vi "PowerElectrodesDlg.vi"(8 "error in":errorcluster caption="error out") -> (0 "error out":errorcluster)   [LabVIEW 2014, in "PowerElectrodes.lvlib"]
uses:
  PowerElectrodes.lvlib
  <vilib>/Utility/miscctls.llb/LVRowAndColumnTypeDef.ctl
  DataBase/DataBase.lvlib
  DetectElecrodes/DetectElectros.lvlib
panel:
  in  "退出":bool
  in  "删除":bool
  in  "修改":bool
  in  "新增":bool
  in  "供电电极管理":i32(listbox)
  in  "OK":bool
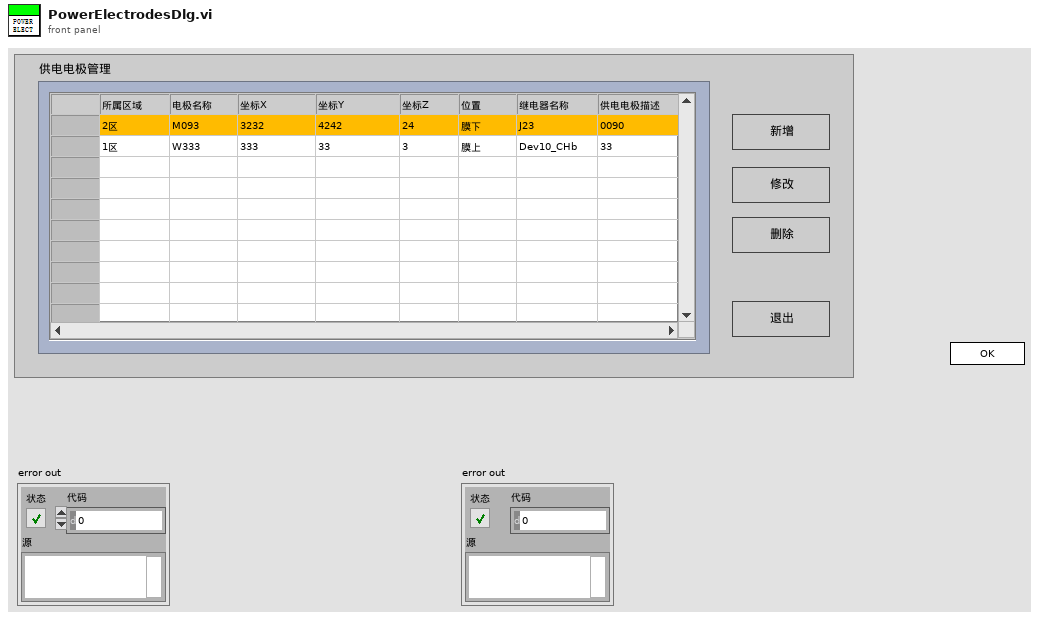
[diagram p1: front panel]
types:
  T1 = enum32{"invalid app kind", "Development System", "Run Time System", "Student Edition", "Embedded LabVIEW", "Evaluation", "Custom"}
  T2 = enum32{"Invalid", "Standard", "Closed", "Hidden", "Minimized", "Maximized"}
  T3 = typedef "LVPoint32TypeDef.ctl" = cluster{"Horizontal":i32, "Vertical":i32}
  T4 = typedef "LVRowAndColumnTypeDef.ctl" = cluster{"Row":i32, "Column":i32}
  T5 = cluster{"Core":cluster{"Current VI Reference":refnum<vi>, "Close Panel on Exit?":bool}, "Your Boolean data":bool, "Your string data":string, "DataP_Init":cluster{i32, "电极名称":string, "区域名称":string, "坐标X":string, "坐标Y":string, "坐标Z":string, "电极位置":string, "继电器名称":string, "继电器极性":string, "电极描述":string}, "行列编号":T4}
  T6 = cluster{i32, "电极名称":string, "区域名称":string, "坐标X":string, "坐标Y":string, "坐标Z":string, "电极位置":string, "继电器名称":string, "继电器极性":string, "电极描述":string}
  T7 = cluster{"Current VI Reference":refnum<vi>, "Close Panel on Exit?":bool}
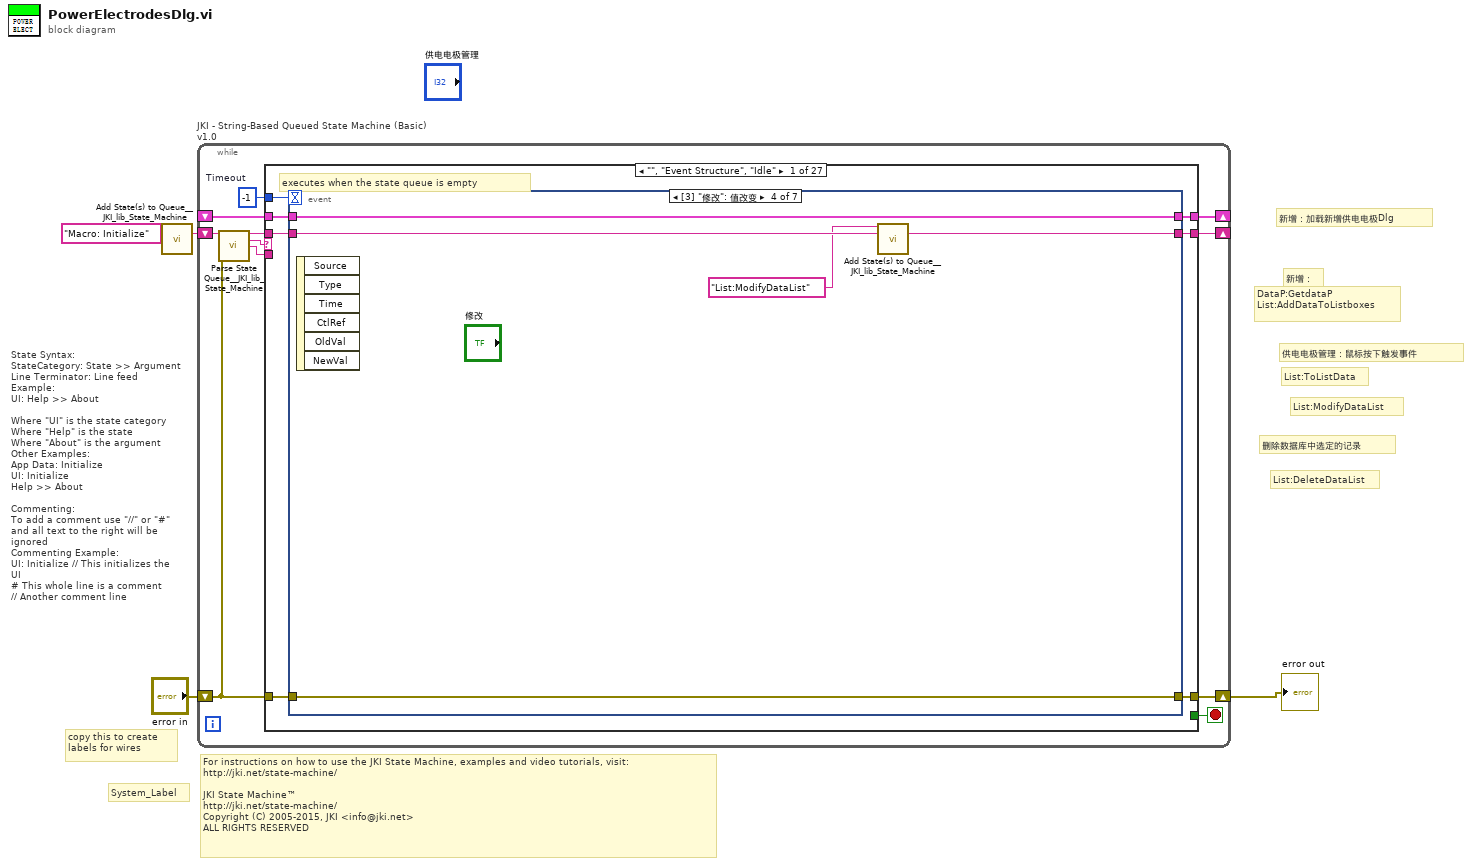
[diagram p0: block diagram]
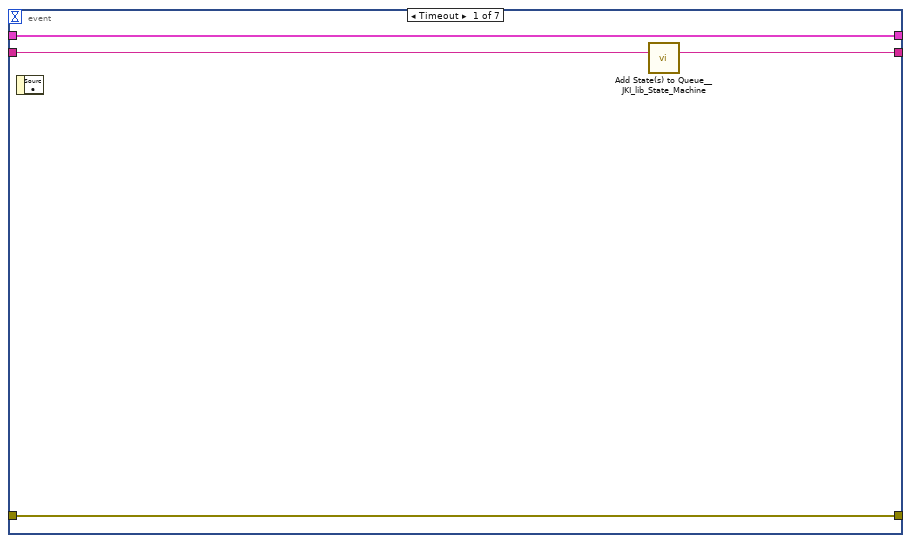
[diagram p2: hidden frame]
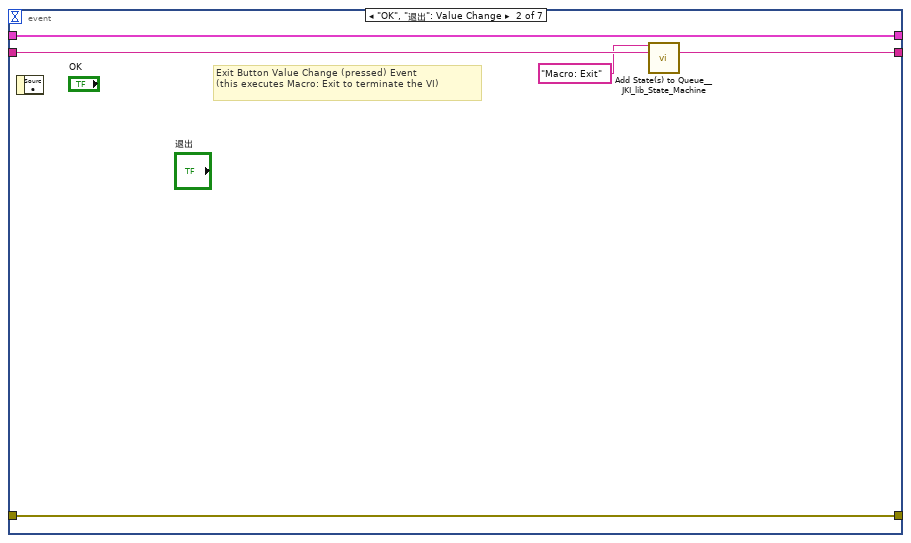
[diagram p3: hidden frame]
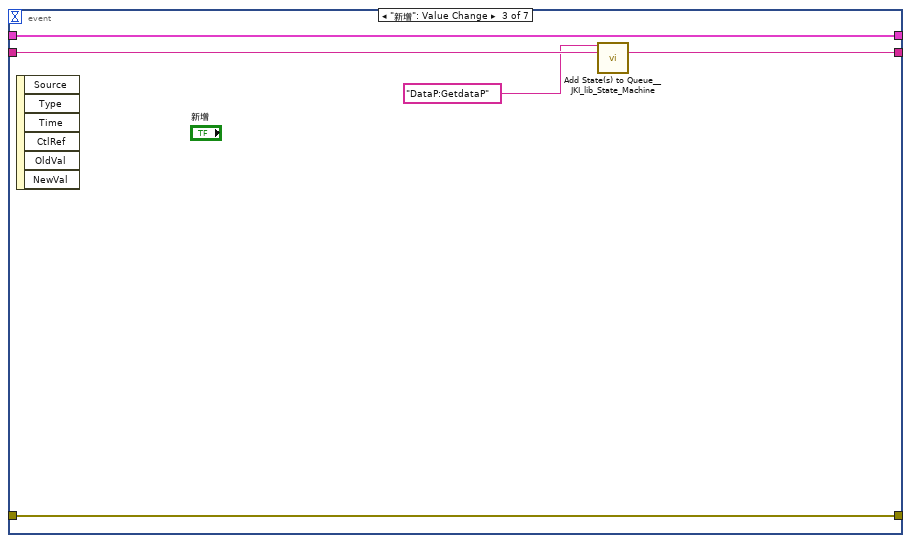
[diagram p4: hidden frame]
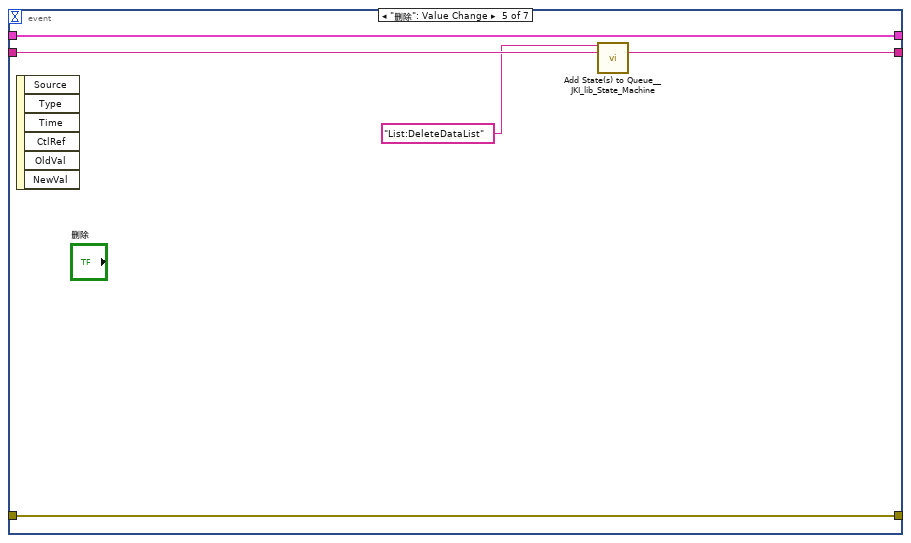
[diagram p5: hidden frame]
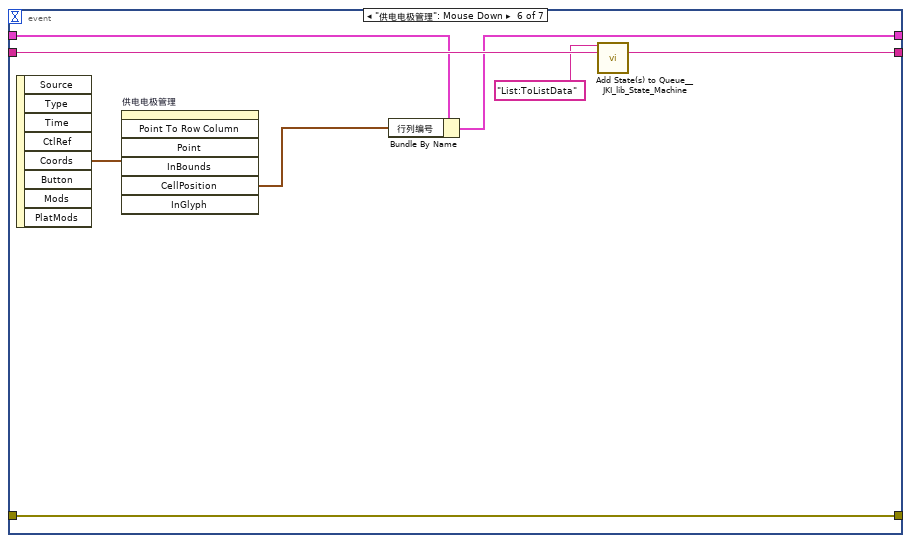
[diagram p6: hidden frame]
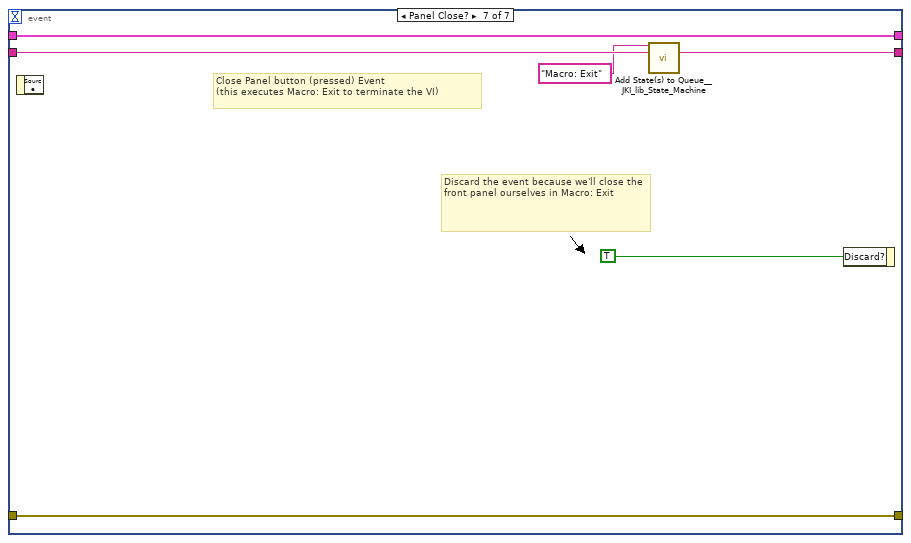
[diagram p7: hidden frame]
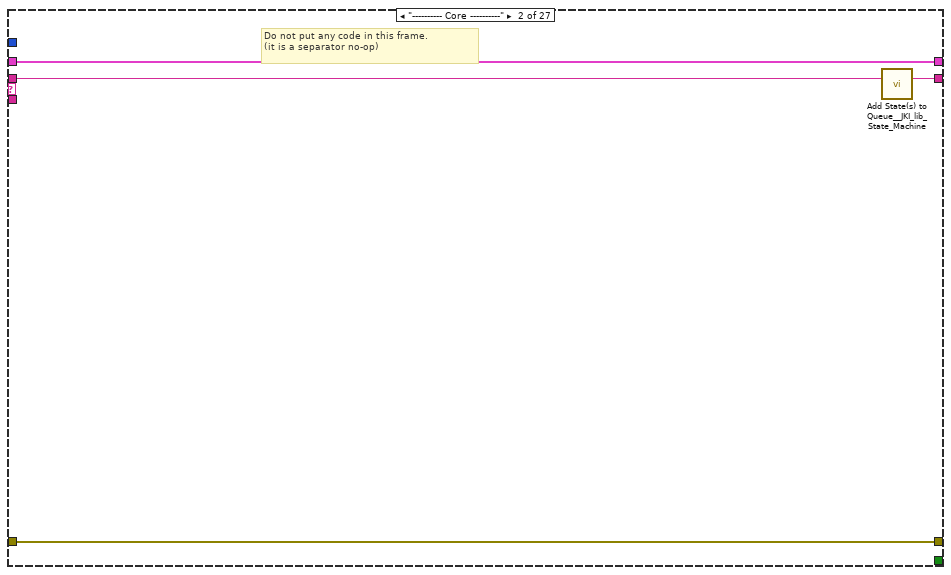
[diagram p8: hidden frame]
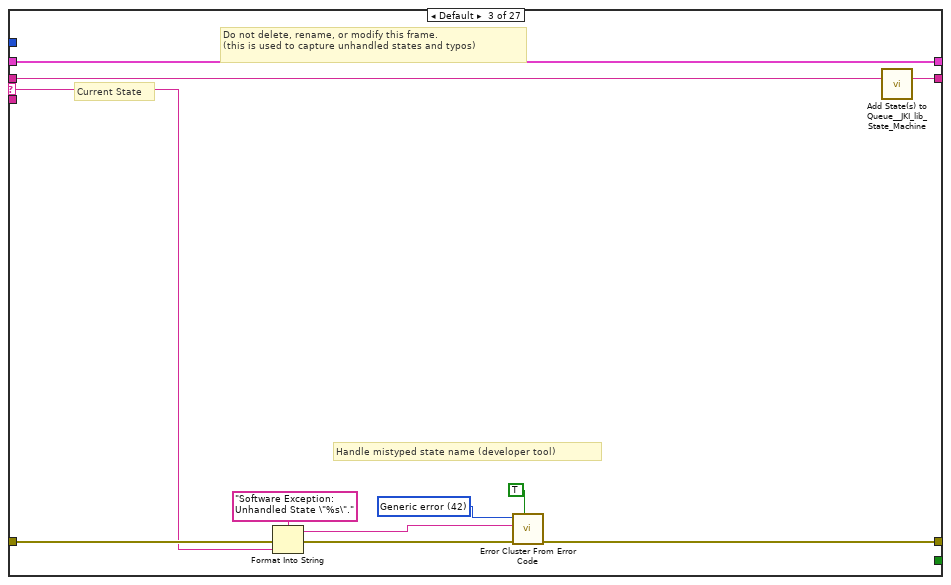
[diagram p9: hidden frame]
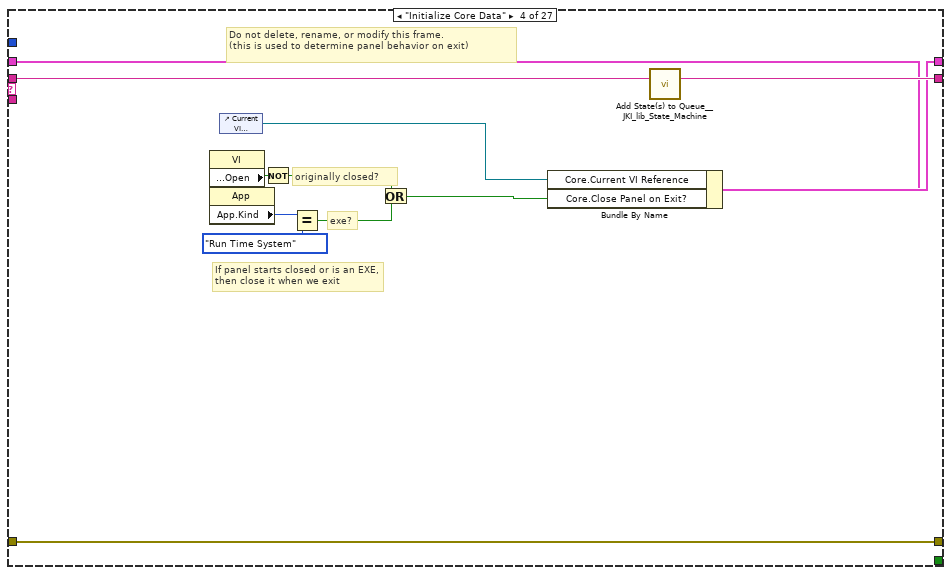
[diagram p10: hidden frame]
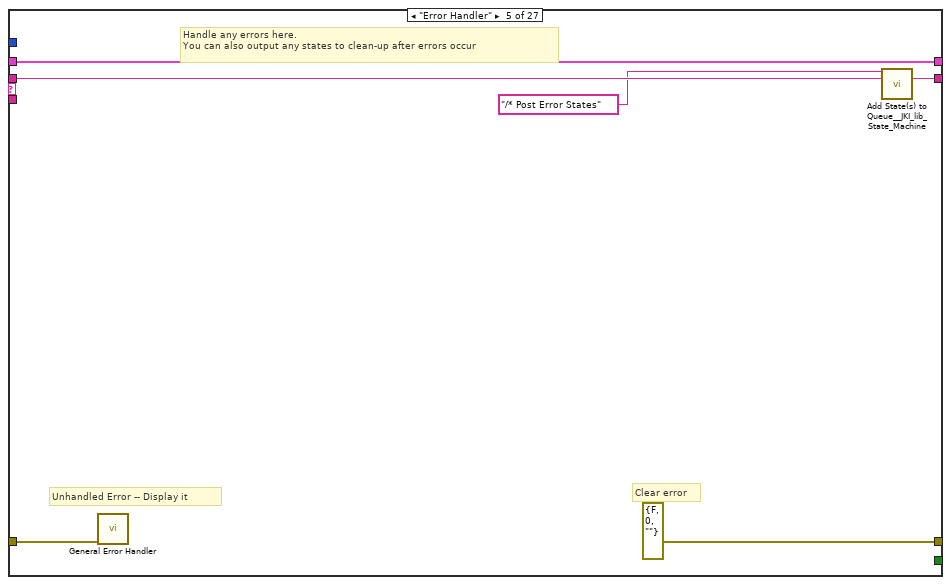
[diagram p11: hidden frame]
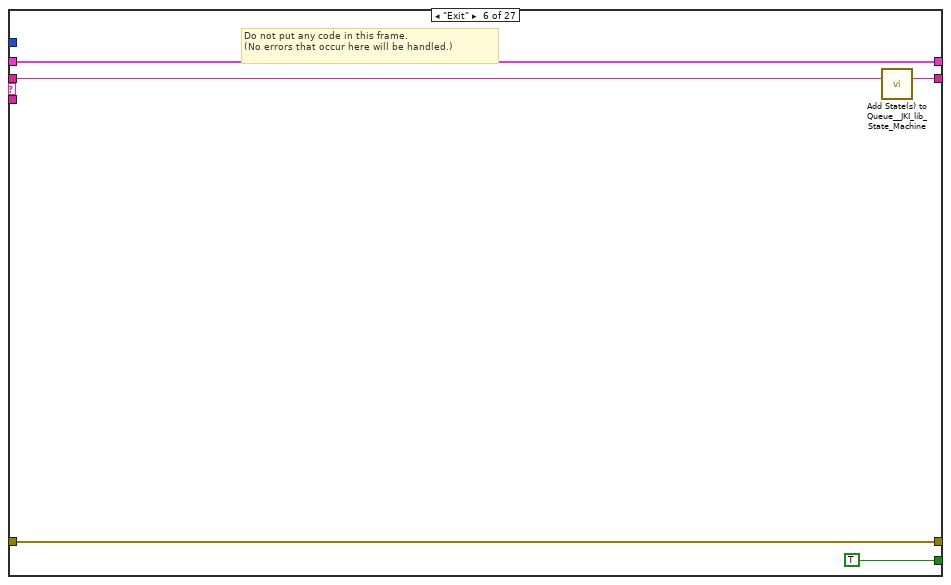
[diagram p12: hidden frame]
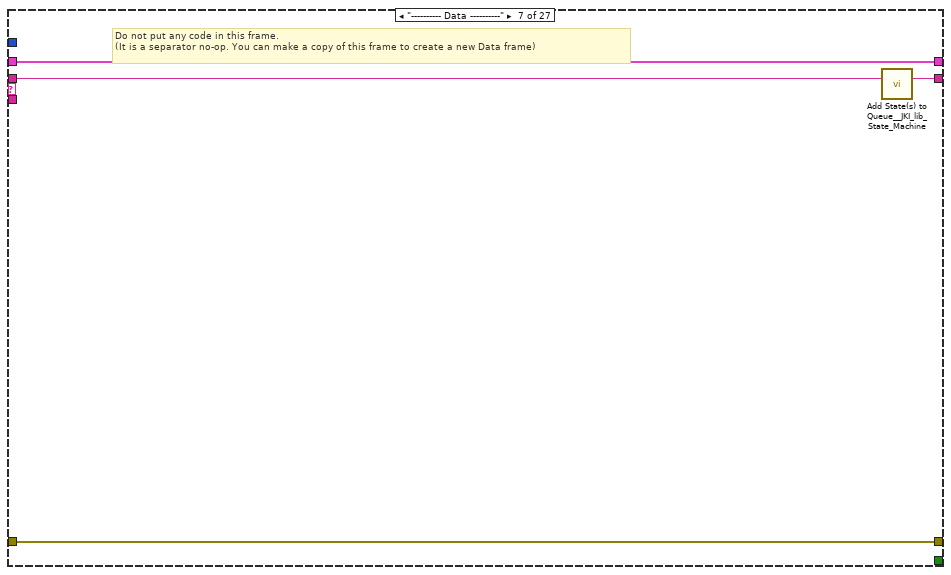
[diagram p13: hidden frame]
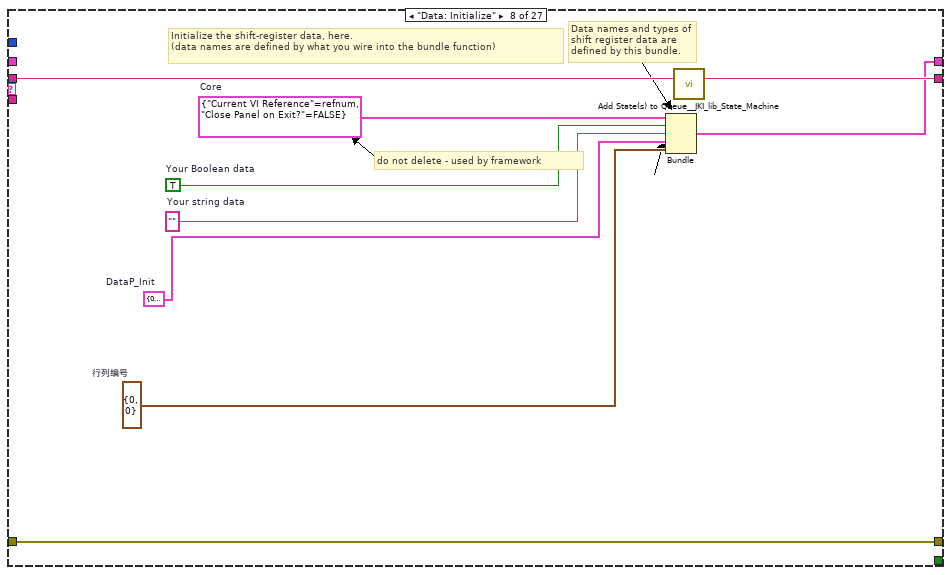
[diagram p14: hidden frame]
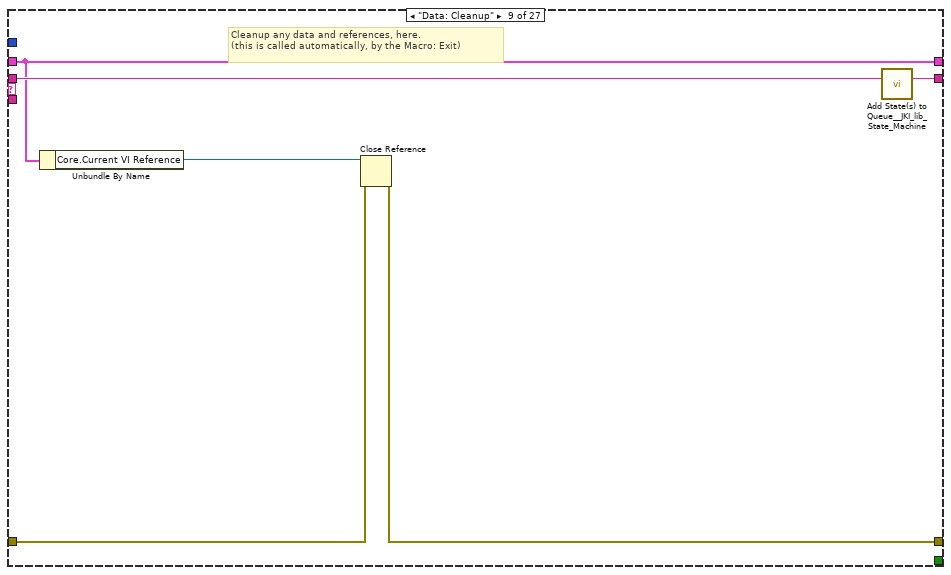
[diagram p15: hidden frame]
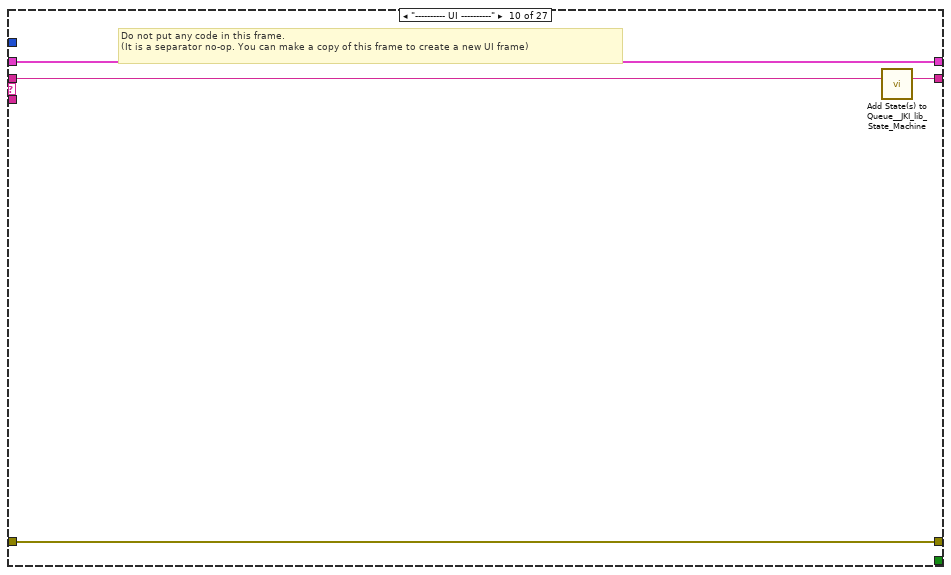
[diagram p16: hidden frame]
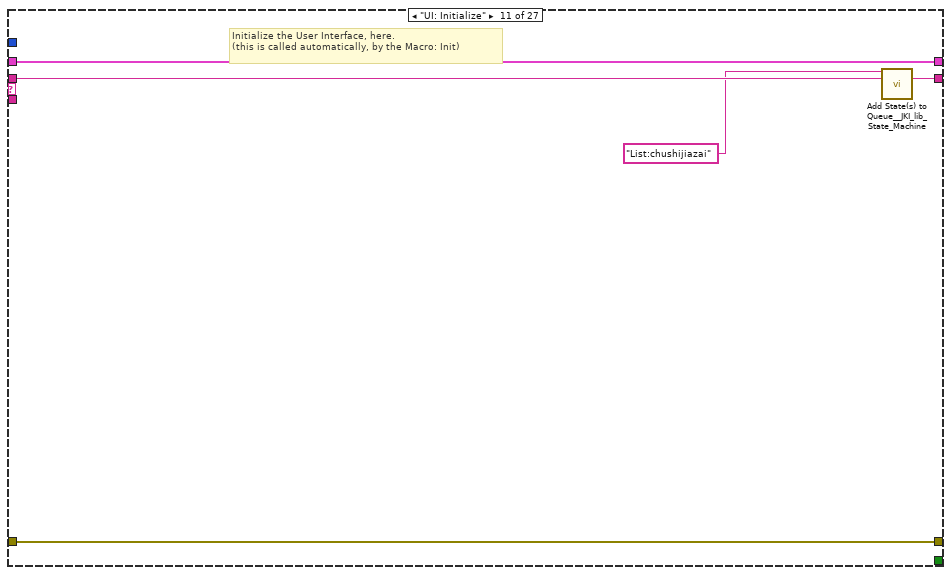
[diagram p17: hidden frame]
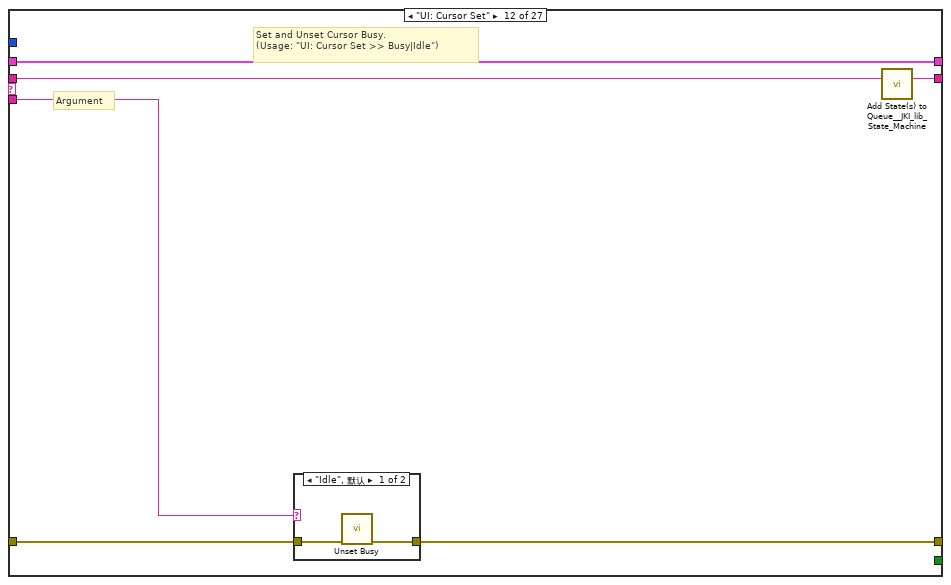
[diagram p18: hidden frame]
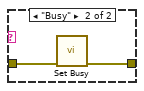
[diagram p19: hidden frame]
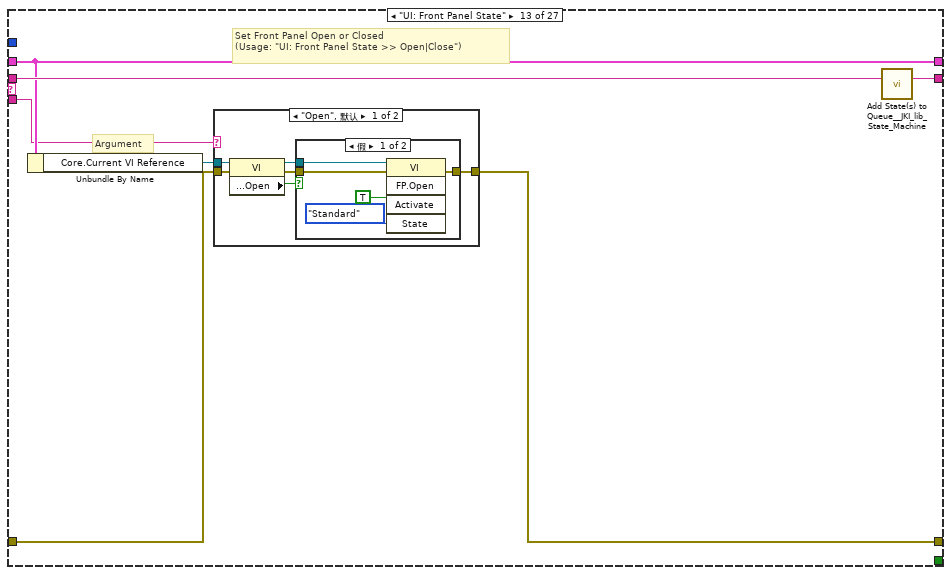
[diagram p20: hidden frame]
diagram:
  # "List:DeleteDataList"
  # "删除数据库中选定的记录"
  # "List:ModifyDataList"
  # "List:ToListData"
  # "供电电极管理：鼠标按下触发事件"
  # "新增："
  # "DataP:GetdataP\nList:AddDataToListboxes"
  # "新增：加载新增供电电极Dlg"
  # "For instructions on how to use the JKI State Machine, examples and video tutorials, visit:\nhttp://jki.net/state-machine/\n\nJKI State Machine™\nhttp://jki.net/state-machine/\nCopyright (C) 2005-2015, JKI <info@jki.net>\nALL RIGHTS RESERVED"
  # "State Syntax:\nStateCategory: State >> Argument\nLine Terminator: Line feed\nExample:\nUI: Help >> About\n\nWhere \"UI\" is the state category\nWhere \"Help\" is the state\nWhere \"About\" is the argument\nOther Examples:\nApp Data: Initialize\nUI: Initialize\nHelp >> About\n\nCommenting:\nTo add a comment use \"//\" or \"#\" and all text to the right will be ignored\nCommenting Example:\nUI: Initialize // This initializes the UI\n# This whole line is a comment\n// Another comment line"
  # "copy this to create labels for wires"
  # "System_Label"
  n1 = call <vilib>:"Add State(s) to Queue__JKI_lib_State_Machine.vi"("State(s) in (\"\")"="Macro: Initialize") -> ("States Out"=w4:string)  [unwired: 14 in]
  n2 = while "JKI - String-Based Queued State Machine (Basic) v1.0" {
    shift-right: [w8] -> _
    shift-left: _ -> [w7]
    shift-right: [w11] -> w2
    shift-left: "error in" -> [w5]
    shift-right: [w10] -> _
    shift-left: w4 -> [w12]
    stop <- w9 stop-if-true
    w6 = -1  # Timeout
    n3 = call <vilib>:"Parse State Queue__JKI_lib_State_Machine.vi"("State Queue"=w12, "Error In (no error)"=w5) -> ("Remaining States"=w14:string, "Current State"=w15:string, "Arguments"=w13:string)  [unwired: 11 in]
    n4 = case shown="\"\", \"Event Structure\", \"Idle\"" w15 {
      selector: w15 -> [_ _ w65 _ _ _ _ _ _ _ _ _ _ _ _ _ _ _ _ _ _ _ _ _ _ _ _]
      tunnel: w14 -> [w22 w64 w69 w87 w93 w98 w102 w111 w117 w121 w126 w132 w143 w169 w174 w184 w188 w192 w201 w208 w212 w225 w252 w279 w283 w287 w291]
      tunnel: w13 -> [_ _ _ _ _ _ _ _ _ _ _ w127 w137 _ _ _ _ _ _ _ _ _ _ _ _ _ _]
      tunnel: w7 -> [w20 w61 w67 w78 w90 w96 w99 _ w112 w118 w124 w130 w139 w166 w171 w181 w185 w189 w198 w204 w209 w222 w249 w276 w280 w284 w288]
      tunnel: [w19 w62 w71 w84 errorcluster {"status"=FALSE, "code"=0, "source"=""} ("error out") w95 w100 w108 w113 w119 w123 w128 w140 w167 w172 w182 w186 w190 w199 w206 w210 w223 w250 w277 w281 w285 w289] -> w11
      tunnel: w5 -> [w18 w62 w70 w84 w89 w95 w100 w108 w114 w119 w123 w129 w141 w167 w172 w182 w186 w190 w199 w206 w210 w223 w250 w277 w281 w285 w289]
      tunnel: [w21 w63 w68 w86 w92 w97 w101 w110 w116 w120 w125 w131 w142 w168 w173 w183 w187 w191 w200 w207 w211 w224 w251 w278 w282 w286 w290] -> w10
      tunnel: [_ _ _ _ _ TRUE _ _ _ _ _ _ _ _ _ _ _ _ _ _ _ _ _ _ _ _ _] -> w9
      tunnel: [w17 w61 w67 w85 w90 w96 w99 w109 w112 w118 w124 w130 w139 w166 w171 w181 w185 w189 w198 w203 w209 w222 w249 w276 w280 w284 w288] -> w8
      tunnel: w6 -> [w16 _ _ _ _ _ _ _ _ _ _ _ _ _ _ _ _ _ _ _ _ _ _ _ _ _ _]
      frame "", "Event Structure", "Idle" {
        # "executes when the state queue is empty"
        n5 = event shown="[3] \"修改\": 值改变" {
          selector: _ -> [_ _ _ _ _ _ _]
          dyn-events: _ -> [_ _ _ _ _ _ _]
          timeout: w16 -> [_ _ _ _ _ _ _]
          tunnel: w22 -> [w26 w31 w34 w39 w44 w53 w60]
          tunnel: [w25 w30 w35 w40 w45 w54 w59] -> w21
          tunnel: w20 -> [w23 w28 w36 w41 w46 w49 w57]
          tunnel: [w24 w29 w33 w38 w43 w52 w58] -> w19
          tunnel: w18 -> [w24 w29 w33 w38 w43 w52 w58]
          tunnel: [w23 w28 w36 w41 w46 w48 w57] -> w17
          event Timeout {
            n6 = event-data() -> ()  [unwired: 1 in, 1 out]
            n7 = call <vilib>:"Add State(s) to Queue__JKI_lib_State_Machine.vi"("State(s) in (\"\")"=w26) -> ("States Out"=w25:string)  [unwired: 14 in]
          }
          event "OK", "退出": Value Change {
            # "Exit Button Value Change (pressed) Event\n(this executes Macro: Exit to terminate the VI)"
            n8 = event-data() -> ()  [unwired: 1 in, 1 out]
            n9 = call <vilib>:"Add State(s) to Queue__JKI_lib_State_Machine.vi"("State(s) in Front (\"\")"="Macro: Exit", "State(s) in (\"\")"=w31) -> ("States Out"=w30:string)  [unwired: 13 in]
          }
          event "新增": Value Change {
            n10 = event-data() -> ()  [unwired: 1 in, 6 out]
            n11 = call <vilib>:"Add State(s) to Queue__JKI_lib_State_Machine.vi"("State(s) in Front (\"\")"="DataP:GetdataP", "State(s) in (\"\")"=w34) -> ("States Out"=w35:string)  [unwired: 13 in]
          }
          event "修改": Value Change {
            n12 = event-data() -> ()  [unwired: 1 in, 6 out]
            n13 = call <vilib>:"Add State(s) to Queue__JKI_lib_State_Machine.vi"("State(s) in Front (\"\")"="List:ModifyDataList", "State(s) in (\"\")"=w39) -> ("States Out"=w40:string)  [unwired: 13 in]
          }
          event "删除": Value Change {
            n14 = event-data() -> ()  [unwired: 1 in, 6 out]
            n15 = call <vilib>:"Add State(s) to Queue__JKI_lib_State_Machine.vi"("State(s) in Front (\"\")"="List:DeleteDataList", "State(s) in (\"\")"=w44) -> ("States Out"=w45:string)  [unwired: 13 in]
          }
          event "供电电极管理": Mouse Down {
            n16 = event-data() -> ("Coords"=w51:T3)  [unwired: 1 in, 7 out]
            n17 = invoke on="供电电极管理" class="MCListbox (严格)" method="Point To Row Column"("Point"=w51) -> ("CellPosition"=w50:T4)  [unwired: 6 in, 6 out]
            n18 = Bundle By Name(cluster=w49, "行列编号"=w50) -> (w48:T5)
            n19 = call <vilib>:"Add State(s) to Queue__JKI_lib_State_Machine.vi"("State(s) in Front (\"\")"="List:ToListData", "State(s) in (\"\")"=w53) -> ("States Out"=w54:string)  [unwired: 13 in]
          }
          event Panel Close? {
            # "Discard the event because we'll close the front panel ourselves in Macro: Exit"
            # "Close Panel button (pressed) Event\n(this executes Macro: Exit to terminate the VI)"
            n20 = event-data() -> ()  [unwired: 1 in, 1 out]
            n21 = call <vilib>:"Add State(s) to Queue__JKI_lib_State_Machine.vi"("State(s) in Front (\"\")"="Macro: Exit", "State(s) in (\"\")"=w60) -> ("States Out"=w59:string)  [unwired: 13 in]
            n22 = event-data("Discard?"=TRUE) -> ()  [unwired: 1 in, 1 out]
          }
        }
      }
      frame "---------- Core ----------" {
        # "Do not put any code in this frame.\n(it is a separator no-op)"
        n23 = call <vilib>:"Add State(s) to Queue__JKI_lib_State_Machine.vi"("State(s) in (\"\")"=w64) -> ("States Out"=w63:string)  [unwired: 14 in]
      }
      frame Default {
        w74 = 42 items=["No error", "Argument error", "Memory is full", "Out of zone", "End of file", "File already open", "Generic file I/O error", "File not found", "File permission error", "Disk is full", "Duplicate path", "Too many files open", "System feature not enabled", "Resource file not found", "Cannot add resource", "Resource not found", "Image not found", "Image memory error", "Pen does not exist", "Config type invalid", "Config token not found", "Config parse error", "Config memory error", "Bad external code format", "Bad external code offset", "External code not present", "Null window", "Destroy window error", "Null menu", "Print aborted", "Bad print record", "Print driver error", "Windows error during printing", "Memory error during printing", "Print dialog error", "Generic print error", "Invalid device refnum", "Device not found", "Device parameter error", "Device unit error", "Cannot open device", "Device call aborted", "Generic error", "Cancelled by user", "Object ID too low", "Object ID too high", "Object not in heap", "Unknown heap", "Unknown object (invalid DefProc)", "Unknown object (DefProc not in table)", "Message out of range", "Invalid (null) method", "Unknown message", "Manager call not supported", "Bad address", "Network operation in progress", "Network operation timed out", "Connection is busy", "Network attribute not supported", "Network error", "Address in use", "System out of memory", "Connection aborted", "Connection refused", "Not connected", "Already connected", "Connection closed", "Initialization error (interapplication manager)", "Bad occurrence", "Wait on unbound occurrence handler", "Occurrence queue overflow", "Datalog type conflict", "Unused", "Unrecognized type (interapplication manager)", "Memory corrupt", "Failed to make temporary DLL", "Old CIN version", "Drag socket not found", "Failed to load drop-object", "Failed to register OLE object", "Failed to release OLE object", "Format specifier type mismatch", "Unknown format specifier", "Too few format specifiers", "Too many format specifiers", "Scan failed", "Newer CIN version", "Error converting to variant", "Runtime menu error", "Password tampered", "Variant attribute not found", "Incompatible variant data type", "Event data is not available", "Event Store is not present", "Occurrence is not found", "Event Queue is not created", "Event info is not available", "Refnum passed is NULL", "Error retrieving Class GUID", "Error retrieving CoClass GUID", "Error retrieving TypeLib GUID.", "Bad built application magic bytes.", "Specific driver is different from the specific driver associated with the Logical Name.", "There is no session opened to the class driver.", "Max Error", "MAX - Error with config objects", "MAX - Error loading configuration", "MAX - Group not supported"]
        # "Current State"
        # "Do not delete, rename, or modify this frame.\n(this is used to capture unhandled states and typos)"
        # "Handle mistyped state name (developer tool)"
        n24 = Format Into String(format string="Software Exception: Unhandled State \"%s\"." ("message"), error in=w70, w65) -> (resulting string=w73:string, error out=w72:errorcluster)  [unwired: 1 in]
        n25 = call <vilib>:"Error Cluster From Error Code.vi"("show call chain? (False)"=TRUE, "error in (no error)"=w72, "error message (\"\")"=w73, "error code (0)"=w74) -> ("error out"=w71:errorcluster)  [unwired: 5 in]
        n26 = call <vilib>:"Add State(s) to Queue__JKI_lib_State_Machine.vi"("State(s) in (\"\")"=w69) -> ("States Out"=w68:string)  [unwired: 14 in]
      }
      frame "Initialize Core Data" {
        # "Do not delete, rename, or modify this frame.\n(this is used to determine panel behavior on exit)"
        # "originally closed?"
        # "exe?"
        # "If panel starts closed or is an EXE, then close it when we exit"
        n27 = property class="VI"() -> ("Front Panel.Open"=w83:bool)  [unwired: 2 in, 2 out]
        n28 = property class="App"() -> ("App.Kind"=w82:T1)  [unwired: 2 in, 2 out]
        n29 = control-ref of="Current VI Reference"() -> (w76:refnum<vi>)
        n30 = Not(x=w83) -> (.not. x?=w80:bool)
        n31 = Equal?(x=w82, y=T1."Run Time System" ("Application:Kind")) -> (x = y?=w79:bool)
        n32 = Or(x=w80, y=w79) -> (x .or. y?=w77:bool)
        n33 = Bundle By Name(cluster=w78, "Core.Current VI Reference"=w76, "Core.Close Panel on Exit?"=w77) -> (w85:T5)
        n34 = call <vilib>:"Add State(s) to Queue__JKI_lib_State_Machine.vi"("State(s) in (\"\")"=w87) -> ("States Out"=w86:string)  [unwired: 14 in]
      }
      frame "Error Handler" {
        # "Unhandled Error -- Display it"
        # "Handle any errors here.\nYou can also output any states to clean-up after errors occur"
        # "Clear error"
        n35 = call <vilib>:"General Error Handler.vi"("error in (no error)"=w89) -> ()  [unwired: 10 in, 5 out]
        n36 = call <vilib>:"Add State(s) to Queue__JKI_lib_State_Machine.vi"("State(s) in Front (\"\")"="/* Post Error States", "State(s) in (\"\")"=w93) -> ("States Out"=w92:string)  [unwired: 13 in]
      }
      frame "Exit" {
        # "Do not put any code in this frame.\n(No errors that occur here will be handled.)"
        n37 = call <vilib>:"Add State(s) to Queue__JKI_lib_State_Machine.vi"("State(s) in (\"\")"=w98) -> ("States Out"=w97:string)  [unwired: 14 in]
      }
      frame "---------- Data ----------" {
        # "Do not put any code in this frame.\n(It is a separator no-op. You can make a copy of this frame to create a new Data frame)"
        n38 = call <vilib>:"Add State(s) to Queue__JKI_lib_State_Machine.vi"("State(s) in (\"\")"=w102) -> ("States Out"=w101:string)  [unwired: 14 in]
      }
      frame "Data: Initialize" {
        w103 = T4 {"Row"=0, "Column"=0}  # 行列编号
        w104 = T6 {0, "电极名称"="", "区域名称"="", "坐标X"="", "坐标Y"="", "坐标Z"="", "电极位置"="", "继电器名称"="", "继电器极性"="", "电极描述"=""}  # DataP_Init
        w105 = T7 {"Current VI Reference"=refnum, "Close Panel on Exit?"=FALSE}  # Core
        w107 = TRUE  # Your Boolean data
        w106 = ""  # Your string data
        # "do not delete - used by framework"
        # "Data names and types of shift register data are defined by this bundle."
        # "Initialize the shift-register data, here.\n(data names are defined by what you wire into the bundle function)"
        n39 = Bundle("Core"=w105, "Your Boolean data"=w107, "Your string data"=w106, "DataP_Init"=w104, "行列编号"=w103) -> (w109:T5)  [unwired: 1 in]
        n40 = call <vilib>:"Add State(s) to Queue__JKI_lib_State_Machine.vi"("State(s) in (\"\")"=w111) -> ("States Out"=w110:string)  [unwired: 14 in]
      }
      frame "Data: Cleanup" {
        # "Cleanup any data and references, here.\n(this is called automatically, by the Macro: Exit)"
        n41 = Unbundle By Name(w112) -> ("Core.Current VI Reference"=w115:refnum<vi>)
        n42 = Close Reference(reference=w115, error in (no error)=w114) -> (error out=w113:errorcluster)
        n43 = call <vilib>:"Add State(s) to Queue__JKI_lib_State_Machine.vi"("State(s) in (\"\")"=w117) -> ("States Out"=w116:string)  [unwired: 14 in]
      }
      frame "---------- UI ----------" {
        # "Do not put any code in this frame.\n(It is a separator no-op. You can make a copy of this frame to create a new UI frame)"
        n44 = call <vilib>:"Add State(s) to Queue__JKI_lib_State_Machine.vi"("State(s) in (\"\")"=w121) -> ("States Out"=w120:string)  [unwired: 14 in]
      }
      frame "UI: Initialize" {
        # "Initialize the User Interface, here.\n(this is called automatically, by the Macro: Init)"
        n45 = call <vilib>:"Add State(s) to Queue__JKI_lib_State_Machine.vi"("State(s) in Front (\"\")"="List:chushijiazai", "State(s) in (\"\")"=w126) -> ("States Out"=w125:string)  [unwired: 13 in]
      }
      frame "UI: Cursor Set" {
        # "Argument"
        # "Set and Unset Cursor Busy.\n(Usage: \"UI: Cursor Set >> Busy|Idle\")"
        n46 = case shown="\"Idle\", 默认" w127 {
          tunnel: w129 -> [w134 w136]
          tunnel: [w133 w135] -> w128
          frame "Idle", Default {
            n47 = call <vilib>:"Unset Busy.vi"("error in (no error)"=w134) -> ("error out"=w133:errorcluster)  [unwired: 10 in]
          }
          frame "Busy" {
            n48 = call <vilib>:"Set Busy.vi"("error in (no error)"=w136) -> ("error out"=w135:errorcluster)  [unwired: 9 in, 1 out]
          }
        }
        n49 = call <vilib>:"Add State(s) to Queue__JKI_lib_State_Machine.vi"("State(s) in (\"\")"=w132) -> ("States Out"=w131:string)  [unwired: 14 in]
      }
      frame "UI: Front Panel State" {
        # "Argument"
        # "Set Front Panel Open or Closed\n(Usage: \"UI: Front Panel State >> Open|Close\")"
        n50 = Unbundle By Name(w139) -> ("Core.Current VI Reference"=w138:refnum<vi>)
        n51 = case shown="\"Open\", 默认" w137 {
          tunnel: w141 -> [w147 w160]
          tunnel: [w149 w161] -> w140
          tunnel: w138 -> [w148 w158]
          frame "Open", Default {
            n52 = property class="VI"(reference=w148, error in=w147) -> (reference out=w145:refnum<vi>, error out=w146:errorcluster, "Front Panel.Open"=w144:bool)
            n53 = case shown="假" w144 {
              tunnel: [w152 w155] -> w149
              tunnel: w146 -> [w151 w155]
              tunnel: w145 -> [w150 _]
              frame False {
                n54 = invoke class="VI" method="FP.Open"(reference=w150, error in=w151, "Activate"=TRUE, "State"=T2."Standard") -> (error out=w152:errorcluster)  [unwired: 1 in, 4 out]
              }
              frame True {
              }
            }
          }
          frame "Close" {
            n55 = property class="VI"(reference=w158, error in=w160) -> (reference out=w157:refnum<vi>, error out=w159:errorcluster, "Front Panel.Open"=w156:bool)
            n56 = case shown="真" w156 {
              tunnel: [w162 w165] -> w161
              tunnel: w159 -> [w162 w164]
              tunnel: w157 -> [_ w163]
              frame False {
              }
              frame True {
                n57 = invoke class="VI" method="FP.Close"(reference=w163, error in=w164) -> (error out=w165:errorcluster)  [unwired: 1 in, 2 out]
              }
            }
          }
        }
        n58 = call <vilib>:"Add State(s) to Queue__JKI_lib_State_Machine.vi"("State(s) in (\"\")"=w143) -> ("States Out"=w142:string)  [unwired: 14 in]
      }
      frame "---------- Macro ----------" {
        # "Do not put any code in this frame.\n(It is a separator no-op. You can make a copy of this frame to create a new Macro frame)"
        n59 = call <vilib>:"Add State(s) to Queue__JKI_lib_State_Machine.vi"("State(s) in (\"\")"=w169) -> ("States Out"=w168:string)  [unwired: 14 in]
      }
      frame "Macro: Initialize" {
        w170 = "Data: Initialize\nInitialize Core Data\nUI: Initialize\nUI: Front Panel State >> Open"  # Data: Initialize Initialize Core Data UI: Initialize UI: Front Panel State >> Open
        # "Initialization Macro\n(This is called once, when the VI starts)"
        n60 = call <vilib>:"Add State(s) to Queue__JKI_lib_State_Machine.vi"("State(s) in Front (\"\")"=w170, "State(s) in (\"\")"=w174) -> ("States Out"=w173:string)  [unwired: 13 in]
      }
      frame "Macro: Exit" {
        # "Exit Macro\n(This is called once, when the VI exits)"
        n61 = Unbundle By Name(w181) -> ("Core.Close Panel on Exit?"=w180:bool)
        n62 = Select(t="UI: Front Panel State >> Close", s=w180, f="") -> (s? t:f=w177:string)
        n63 = call <vilib>:"Add State(s) to Queue__JKI_lib_State_Machine.vi"("State(s) in (\"\")"=w177, "State(s) at Back (\"\")"="Data: Cleanup\nExit") -> ("States Out"=w175:string)  [unwired: 13 in]
        n64 = call <vilib>:"Add State(s) to Queue__JKI_lib_State_Machine.vi"("State(s) in Front (\"\")"=w175, "State(s) in (\"\")"=w184) -> ("States Out"=w183:string)  [unwired: 13 in]
      }
      frame "-----------DataP-----------" {
        # "Template Separator\n(You can make a copy of, or modify, this frame)"
        n65 = call <vilib>:"Add State(s) to Queue__JKI_lib_State_Machine.vi"("State(s) in (\"\")"=w188) -> ("States Out"=w187:string)  [unwired: 14 in]
      }
      frame "List:ToListData" {
        # "Template Separator\n(You can make a copy of, or modify, this frame)"
        n66 = call <vilib>:"Add State(s) to Queue__JKI_lib_State_Machine.vi"("State(s) in (\"\")"=w192) -> ("States Out"=w191:string)  [unwired: 14 in]
      }
      frame "List:DeleteDataList" {
        # "select power_electrodes_Id from t_power_electrodes  limit %s,1"
        # "Template Separator\n(You can make a copy of, or modify, this frame)"
        n67 = Unbundle By Name(w198) -> ("行列编号.Row"=w196:i32)
        n68 = Number To Decimal String(number=w196) -> (decimal integer string=w195:string)  [unwired: 1 in]
        n69 = Format Into String(format string="delete from t_power_electrodes where power_electrodes_id =(select tp.power_electrodes_id from \n(select power_electrodes_id from t_power_electrodes  limit %s,1) tp);", w195) -> (resulting string=w194:string)  [unwired: 2 in, 1 out]
        n70 = call "deleteData.vi"("SQL query"=w194) -> ()  [unwired: 10 in, 1 out]
        n71 = call <vilib>:"Add State(s) to Queue__JKI_lib_State_Machine.vi"("State(s) in Front (\"\")"="List:AddDataToListboxes", "State(s) in (\"\")"=w201) -> ("States Out"=w200:string)  [unwired: 13 in]
      }
      frame "DataP:GetdataP" {
        # "Template Separator\n(You can make a copy of, or modify, this frame)"
        n72 = call "New_Power_ElectrodesDlg.vi"() -> ("DataP"=w205:T6)  [unwired: 10 in, 1 out]
        n73 = Bundle By Name(cluster=w204, "DataP_Init"=w205) -> (w203:T5)
        n74 = call <vilib>:"Add State(s) to Queue__JKI_lib_State_Machine.vi"("State(s) in Front (\"\")"="List:AddDataToListboxes", "State(s) in (\"\")"=w208) -> ("States Out"=w207:string)  [unwired: 13 in]
      }
      frame "----------List-------" {
        # "Template Separator\n(You can make a copy of, or modify, this frame)"
        n75 = call <vilib>:"Add State(s) to Queue__JKI_lib_State_Machine.vi"("State(s) in (\"\")"=w212) -> ("States Out"=w211:string)  [unwired: 14 in]
      }
      frame "List:ModifyDataList" {
        # "Template Separator\n(You can make a copy of, or modify, this frame)"
        n76 = Unbundle By Name(w222) -> ("行列编号.Row"=w220:i32)
        n77 = Number To Decimal String(number=w220) -> (decimal integer string=w219:string)  [unwired: 1 in]
        n78 = Format Into String(format string="select *from t_power_electrodes limit %s,1", w219) -> (resulting string=w218:string)  [unwired: 2 in, 1 out]
        n79 = call "SelectData.vi"("SQL query"=w218) -> ("recordset data"=w217:variant[][])  [unwired: 7 in, 1 out]
        n80 = call "ReadDataFromDatabase.vi"("长度"=10, "index"=0, "recordset data"=w217) -> ("一行记录"=w214:string[])  [unwired: 7 in, 1 out]
        n81 = call "Modify_Power_ElectrodesDlg.vi"("一行记录"=w214) -> ()  [unwired: 8 in, 1 out]
        n82 = call <vilib>:"Add State(s) to Queue__JKI_lib_State_Machine.vi"("State(s) in Front (\"\")"="List:AddDataToListboxes", "State(s) in (\"\")"=w225) -> ("States Out"=w224:string)  [unwired: 13 in]
      }
      frame "List:AddDataToListboxes" {
        w238 = 1 ("索引")
        # "从数据库中更新List中数据"
        # "从数据库中获取再在List中显示，这样更新比较好"
        # "Template Separator\n(You can make a copy of, or modify, this frame)"
        n83 = call "SelectData.vi"("SQL query"="select *from t_power_electrodes") -> ("recordset data"=w247:variant[][])  [unwired: 7 in, 1 out]
        n84 = call "ReadDataFromDatabase.vi"("长度"=9, "index"=1, "recordset data"=w247) -> ("所有记录"=w234:string[][])  [unwired: 7 in, 1 out]
        n85 = Array Subset(array=w234, index (col)=w238, length (col)=w238) -> (w236:string[][])  [unwired: 2 in]
        n86 = Array Subset(array=w234, index (col)=0 ("索引"), length (col)=1 ("长度")) -> (w240:string[][])  [unwired: 2 in]
        n87 = Array Subset(array=w234, index (col)=2 ("索引")) -> (w241:string[][])  [unwired: 3 in]
        n88 = Array Subset(array=w234, index (col)=8, length (col)=1 ("索引")) -> (w230:string[][])  [unwired: 2 in]
        n89 = Insert Into Array(array=w241, index (col)=0 ("禁用的索引 (列)"), new element=w240) -> (w237:string[][])  [unwired: 1 in]
        n90 = Insert Into Array(array=w237, index (col)=0 ("禁用的索引 (列)"), new element=w236) -> (w231:string[][])  [unwired: 1 in]
        n91 = Insert Into Array(array=w231, index (col)=7, new element=w230) -> (w228:string[][])  [unwired: 1 in]
        n92 = Array Subset(array=w228, length (col)=8) -> (w226:string[][])  [unwired: 3 in]
        n93 = property on="供电电极管理" class="MCListbox (严格)"("ItemNames"=w226) -> ()  [unwired: 2 in, 2 out]
        n94 = call <vilib>:"Add State(s) to Queue__JKI_lib_State_Machine.vi"("State(s) in (\"\")"=w252) -> ("States Out"=w251:string)  [unwired: 14 in]
      }
      frame "List:chushijiazai" {
        w265 = 1 ("索引")
        # "从数据库中更新List中数据"
        # "从数据库中获取再在List中显示，这样更新比较好"
        # "Template Separator\n(You can make a copy of, or modify, this frame)"
        n95 = call "SelectData.vi"("SQL query"="select *from t_power_electrodes") -> ("recordset data"=w274:variant[][])  [unwired: 7 in, 1 out]
        n96 = call "ReadDataFromDatabase.vi"("长度"=9, "index"=1, "recordset data"=w274) -> ("所有记录"=w261:string[][])  [unwired: 7 in, 1 out]
        n97 = Array Subset(array=w261, index (col)=w265, length (col)=w265) -> (w263:string[][])  [unwired: 2 in]
        n98 = Array Subset(array=w261, index (col)=0 ("索引"), length (col)=1 ("长度")) -> (w267:string[][])  [unwired: 2 in]
        n99 = Array Subset(array=w261, index (col)=2 ("索引")) -> (w268:string[][])  [unwired: 3 in]
        n100 = Array Subset(array=w261, index (col)=8, length (col)=1 ("索引")) -> (w257:string[][])  [unwired: 2 in]
        n101 = Insert Into Array(array=w268, index (col)=0 ("禁用的索引 (列)"), new element=w267) -> (w264:string[][])  [unwired: 1 in]
        n102 = Insert Into Array(array=w264, index (col)=0 ("禁用的索引 (列)"), new element=w263) -> (w258:string[][])  [unwired: 1 in]
        n103 = Insert Into Array(array=w258, index (col)=7, new element=w257) -> (w255:string[][])  [unwired: 1 in]
        n104 = Array Subset(array=w255, length (col)=8) -> (w253:string[][])  [unwired: 3 in]
        n105 = property on="供电电极管理" class="MCListbox (严格)"("ItemNames"=w253) -> ()  [unwired: 2 in, 2 out]
        n106 = call <vilib>:"Add State(s) to Queue__JKI_lib_State_Machine.vi"("State(s) in (\"\")"=w279) -> ("States Out"=w278:string)  [unwired: 14 in]
      }
      frame "---------- New Category ----------" {
        # "Template Separator\n(You can make a copy of, or modify, this frame)"
        n107 = call <vilib>:"Add State(s) to Queue__JKI_lib_State_Machine.vi"("State(s) in (\"\")"=w283) -> ("States Out"=w282:string)  [unwired: 14 in]
      }
      frame "New Category: 1" {
        # "Your code here.\n(You can make a copy of, or modify, this frame)"
        n108 = call <vilib>:"Add State(s) to Queue__JKI_lib_State_Machine.vi"("State(s) in (\"\")"=w287) -> ("States Out"=w286:string)  [unwired: 14 in]
      }
      frame "New Category: 2" {
        # "Your code here.\n(You can make a copy of, or modify, this frame)"
        n109 = call <vilib>:"Add State(s) to Queue__JKI_lib_State_Machine.vi"("State(s) in (\"\")"=w291) -> ("States Out"=w290:string)  [unwired: 14 in]
      }
    }
  }
  "error out" <- w2
